vi "pardiso(SubVI).vi"(10 "b":dbl[](array[numeric]), 11 "A":dbl[][](array[numeric])) -> (3 "Wynik":dbl[](array[numeric]))   [LabVIEW 2020]
uses:
  <vilib>/addons/Multicore Analysis and Sparse Matrix/Matrix/_matrix/Dense to Sparse (DBL).vi
  <vilib>/addons/Multicore Analysis and Sparse Matrix/SparseLinAlg/_sparselinalg/PARDISO Advanced Initialization (DBL).vi
  <vilib>/addons/Multicore Analysis and Sparse Matrix/SparseLinAlg/_sparselinalg/PARDISO Advanced Factorization (DBL).vi
  <vilib>/addons/Multicore Analysis and Sparse Matrix/SparseLinAlg/_sparselinalg/PARDISO Advanced Solver (DBL).vi
  <vilib>/addons/Multicore Analysis and Sparse Matrix/SparseLinAlg/_sparselinalg/PARDISO Advanced Cleaning Up (DBL).vi
  <vilib>/addons/Multicore Analysis and Sparse Matrix/SparseLinAlg/NI_MASM_PARDISO.lvlib
  <vilib>/addons/Multicore Analysis and Sparse Matrix/Matrix/NI_MASM_Matrix.lvlib
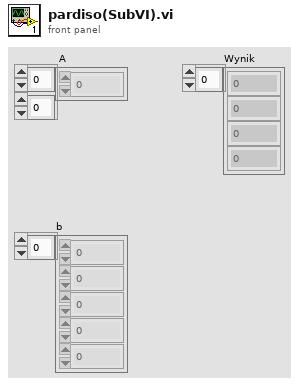
[diagram p1: front panel]
types:
  T1 = typedef "NI_MASM_PARDISO.lvlib/PARDISO Advanced_Solver ID (DBL).ctl" = cluster{"ID":string, "Sparse Matrix":refnum<class "NI_MASM_Sparse_DBL.lvclass">}
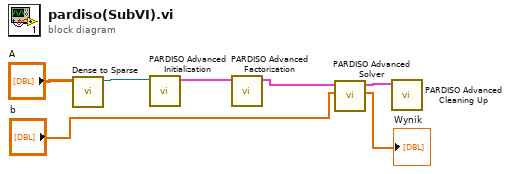
[diagram p0: block diagram]
diagram:
  n1 = call-poly <vilib>:"Dense to Sparse.vi"("Dense Matrix"="A") -> ("Sparse Matrix"=w2:refnum<class "NI_MASM_Sparse_DBL.lvclass">)  [unwired: 9 in, 1 out]
  n2 = call-poly <vilib>:"PARDISO Advanced Initialization.vi"("Input Matrix"=w2) -> ("solver ID"=w3:T1)  [unwired: 8 in, 2 out]
  n3 = call-poly <vilib>:"PARDISO Advanced Factorization.vi"("solver ID in"=w3) -> ("solver ID out"=w4:T1)  [unwired: 8 in, 2 out]
  n4 = call-poly <vilib>:"PARDISO Advanced Solver.vi"("Known Vector"="b", "solver ID in"=w4) -> ("Solution Vector"=→"Wynik":dbl[], "solver ID out"=w6:T1)  [unwired: 6 in, 2 out]
  n5 = call-poly <vilib>:"PARDISO Advanced Cleaning Up.vi"("solver ID"=w6) -> ()  [unwired: 10 in, 1 out]
